vi "get top array index.vi"(8 "error in (no error)":errorcluster, 11 "Array in":refnum<vi>) -> (0 "error out":errorcluster, 1 "last value index":u32, 2 "top index":u32, 3 "Array out":refnum<vi>)   [LabVIEW 2013, in "PID Module editor node.lvclass"]
uses:
  PID Module editor node.lvclass
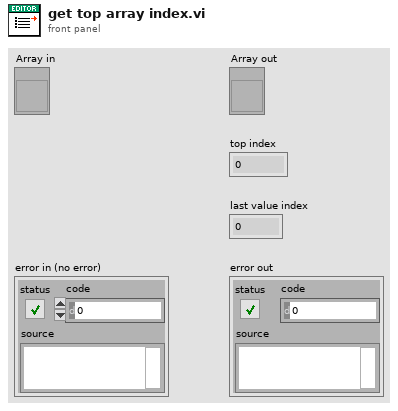
[diagram p1: front panel]
types:
  T1 = cluster{"Loop ID":string, "Tags":cluster{"Setpoint":string, "Process Variable":string, "Output":string}, "Gains":cluster{"P":dbl, "I":dbl, "D":dbl}, "Range":cluster{"High":dbl, "Low":dbl}}[]
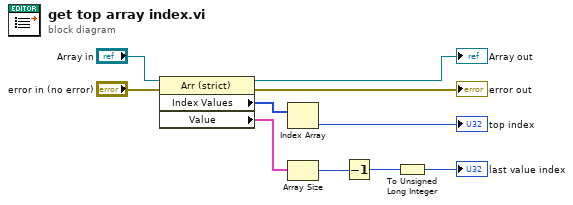
[diagram p0: block diagram]
diagram:
  n1 = property class="Arr (strict)"(reference="Array in", error in="error in (no error)") -> (reference out=→"Array out":refnum<vi>, error out=→"error out":errorcluster, "Index Values"=w10:u32[], "Value"=w4:T1)
  n2 = Index Array(array=w10) -> (element=→"top index":u32)  [unwired: 1 in]
  n3 = Array Size(array=w4) -> (size(s)=w3:i32)
  n4 = Decrement(x=w3) -> (x-1=w2:i32)
  n5 = To Unsigned Long Integer(number=w2) -> (unsigned 32bit integer=→"last value index":u32)
